vi "Stop Core.vi"(10 "final error code":i32, 11 "Sensor Charm View in":refnum<class "Sensor Charm View.lvclass">) -> (3 "Sensor Charm View out":refnum<class "Sensor Charm View.lvclass">)   [LabVIEW 2013, in "Sensor Charm View.lvlib" / "Sensor Charm View.lvclass"]
doc: "(<B>Filename</B>: Actor Framework.lvlib:Actor.lvclass:Stop Core.vi)\n\nDefines what the actor does before it stops. Use the <B>final error code</B> input to determine whether the actor shut down in response to an error.\n\nBy default, this method does nothing. A descendant class may override it to define behavior, such as shutting down any processes the actor initiated in its override of the Actor Core method."
uses:
  Sensor Charm View.lvclass
  <vilib>/ActorFrameworkMVC/View Actor/View Actor.lvclass
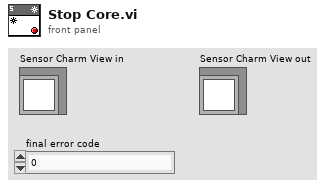
[diagram p1: front panel]
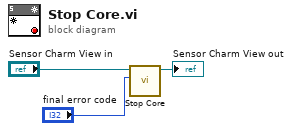
[diagram p0: block diagram]
diagram:
  n1 = call-parent "Stop Core.vi"("final error code"="final error code", "Actor in"="Sensor Charm View in") -> ("Actor out"=→"Sensor Charm View out":refnum<class "Sensor Charm View.lvclass">)  [unwired: 9 in]
